vi "Set Server Address.vi"(10 "Server Address":string, 11 "OOP Server in":refnum<class "HVC4.lvclass">) -> (3 "OOP Server out":refnum<class "HVC4.lvclass">)   [LabVIEW 2019, in "HVC4.lvlib" / "HVC4.lvclass"]
uses:
  HVC4.lvclass
  HVC4.lvclass/HVC4.ctl
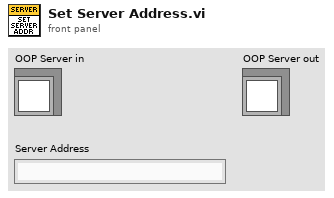
[diagram p1: front panel]
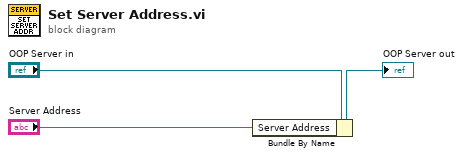
[diagram p0: block diagram]
diagram:
  n1 = Bundle By Name(cluster="OOP Server in", "Server Address"="Server Address") -> (→"OOP Server out":refnum<class "HVC4.lvclass">)
